vi "Parse Menu Items.vi"(8 "error in":errorcluster, 11 "Menu Items":cluster{"Tag":string, "Enabled?":bool}[](array[cluster])) -> (0 "error out":errorcluster, 2 "Item Tags":string[](array[string]), 3 "Item Names":string[](array[string]), 5 "Disabled Tags":string[](array[string]))   [LabVIEW 2020, in "Ballard MIL-STD-1553 System Explorer.lvlib"]
uses:
  Ballard MIL-STD-1553 System Explorer.lvlib
  Shared/Constants.vi
  Shared/Ballard MIL-STD-1553 Shared.lvlib
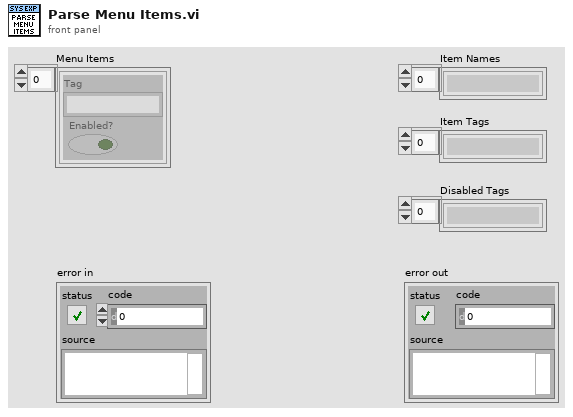
[diagram p1: front panel]
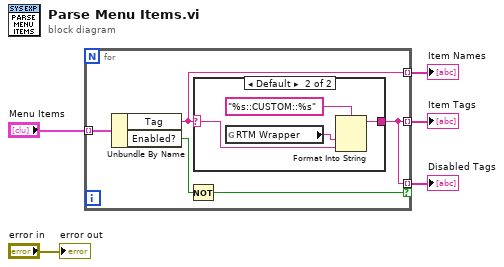
[diagram p0: block diagram]
diagram:
  n1 = for {
    tunnel: "Menu Items" -> [w10] mode=indexing
    tunnel: [w6] -> w1 mode=indexing
    tunnel: [w6] -> w5 mode=indexing if=w8
    tunnel: [w7] -> w2 mode=indexing
    n2 = Unbundle By Name(w10) -> ("Tag"=w7:string, "Enabled?"=w9:bool)
    n3 = Not(x=w9) -> (.not. x?=w8:bool)
    n4 = case shown="Default" w7 {
      selector: w7 -> [w11 w13]
      tunnel: [w11 w12] -> w6
      frame "app_separator" {
      }
      frame Default {
        n5 = global read "Constants.vi" "RTM Wrapper"() -> (w14:string)
        n6 = Format Into String(format string="%s::CUSTOM::%s", w14, w13) -> (resulting string=w12:string)  [unwired: 2 in, 1 out]
      }
    }
  }
  "Disabled Tags" <- w5
  "Item Tags" <- w1
  "Item Names" <- w2
  "error out" <- "error in"
